vi "XML Script - PathToXMLString.vi"(1 "Path":path) -> (0 "Valid XML String (out)":string)   [LabVIEW 2020]
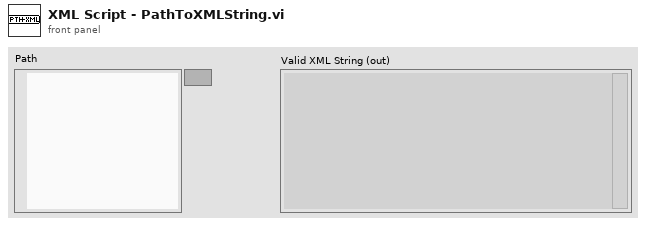
[diagram p1: front panel]
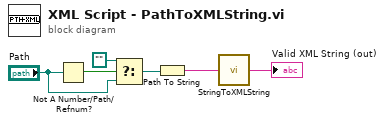
[diagram p0: block diagram]
diagram:
  n1 = Not A Number/Path/Refnum?(number/path/refnum="Path") -> (NaN/Path/Refnum?=w6:bool)
  n2 = Select(t=path "", s=w6, f="Path") -> (s? t:f=w2:path)
  n3 = Path To String(path=w2) -> (string=w3:string)
  n4 = call <vilib>:"StringToXMLString.vi"("String"=w3) -> ("Valid XML String (out)"=→"Valid XML String (out)":string)
